vi "Longer Pump dLSP501 Operation Full Driver.vi"() -> ()   [LabVIEW 2023, in "Longer Pump dLSP501 Series.lvlib"]
uses:
  <instrlib>/Longer Pump dLSP501 Modbus RTU Series/Longer Pump dLSP501 Series.lvlib
  <vilib>/NI/Modbus Library/API/Master/Modbus Master.lvclass
  C:/Program Files/National Instruments/LabVIEW 2023/vi.lib/NI/Modbus Library/API/Modbus API.lvclass
  <instrlib>/Longer Pump dLSP501 Modbus RTU Series/Private/Initialize - Integrated Address.vi
  <vilib>/NI/Modbus Library/API/Modbus API.lvclass
panel:
  in  "Comm Port Control":cluster{"Open Port":bool, "Close Port":bool} caption="串口控制"
  in  "Operation Control":T1 caption="运行控制"
  in  "Fast Run Config":T2={"Drive Force"=80, "Run Speed"=300, "Speed Unit"="rpm", "Full Drive Force Unit"=0} caption="快速运行设置" {"Full Drive Force Unit" items=["%"]; "Run Speed" min=100 max=300 step=1; "Drive Force" min=20 max=100 step=1}
  out "Error Information":string caption="错误信息"
  out "Run Information":string caption="运行信息"
  in  "Syringe Configuration":T3={"Syringe Speicification"=1.0, "Volume Unit"=1, "Syringe Stroke"=57.1513, "Syringe Length Unit"=0} caption="注射器配置" {"Syringe Length Unit" items=["mm"]; "Syringe Stroke" min=0.001; "Volume Unit" items=["mL"=1, "uL"=2]; "Syringe Speicification" min=0.001}
  in  "Run Parameters":T4={"Run Mode"=0, "Volume Value"=1.0, "Volume Unit"=1, "Infuse Flowrate Value"=1.0, "Infuse Flowrate Unit"=1, "Withdraw Flowrate Value"=1.0, "Withdraw Flowrate Unit"=1, "Interval Time 1 Value"=1.0, "Interval Time 1 Unit"=2, "Interval Time 2 Value"=1.0, "Interval Time 2 Unit"=2, "Drive Force"=100, "Drive Force Unit"=0, "Dispensing Times"=1, "Cycles"=1} caption="运行参数" {"Drive Force Unit" items=["%"]; "Dispensing Times" min=1 max=9999; "Interval Time 2 Unit" items=["h", "min", "s"]; "Interval Time 1 Unit" items=["h", "min", "s"]; "Interval Time 2 Value" min=0.001; "Interval Time 1 Value" min=0.001; "Run Mode" items=["灌注模式", "抽取模式", "灌注/抽取模式", "抽取/灌注模式"]; "Withdraw Flowrate Unit" items=["L/min", "mL/min", "uL/min", "nL/min"]; "Withdraw Flowrate Value" min=0.001; "Infuse Flowrate Unit" items=["L/min", "mL/min", "uL/min", "nL/min"]; "Infuse Flowrate Value" min=0.001; "Volume Unit" items=["L", "mL", "uL", "nL"]; "Volume Value" min=0.001}
  out "Error out":errorcluster caption="错误输出"
  in  "Comm Config.":T5={"Address"=1, "Baud Rate"=115200, "Parity"=0} caption="通讯设置" {"Parity" items=["无校验", "奇校验", "偶校验", "标记", "空格"]; "Baud Rate" items=["1200"=1200, "2400"=2400, "9600"=9600, "19200"=19200, "38400"=38400, "57600"=57600, "115200"=115200]}
  in  "VISA resource name":refnum<visa-resource-name>="COM1" caption="VISA资源名"
  in  "Error in":errorcluster caption="错误输入"
  # "设置串口参数后，打开串口，然后进行运行控制。\n1. 全速运行；或设置运行参数、然后启动运行。\n2. 系统定期更新运行状态。"
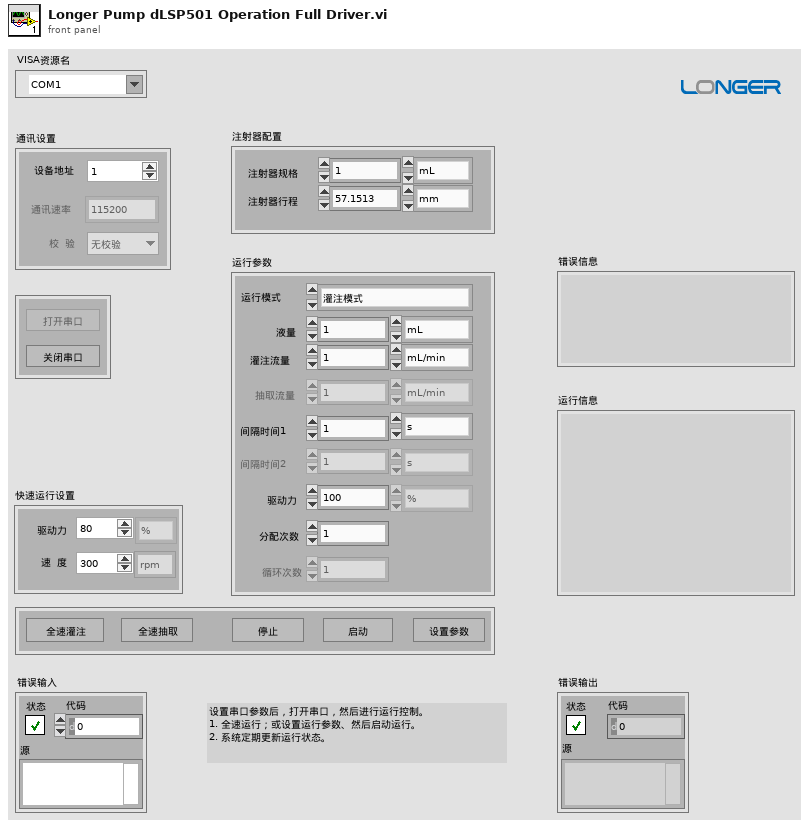
[diagram p1: front panel]
types:
  T1 = cluster{"Set Run Param":bool, "Start Run":bool, "Stop Run":bool, "Fast Infuse":bool, "Fast Withdraw":bool}
  T2 = cluster{"Drive Force":u16, "Run Speed":u16, "Speed Unit":string, "Full Drive Force Unit":u16}
  T3 = cluster{"Syringe Speicification":dbl, "Volume Unit":u16, "Syringe Stroke":dbl, "Syringe Length Unit":u16}
  T4 = cluster{"Run Mode":u16, "Volume Value":dbl, "Volume Unit":u16, "Infuse Flowrate Value":dbl, "Infuse Flowrate Unit":u16, "Withdraw Flowrate Value":dbl, "Withdraw Flowrate Unit":u16, "Interval Time 1 Value":dbl, "Interval Time 1 Unit":u16, "Interval Time 2 Value":dbl, "Interval Time 2 Unit":u16, "Drive Force":u16, "Drive Force Unit":u16, "Dispensing Times":u16, "Cycles":u16}
  T5 = cluster{"Address":u8, "Baud Rate":u32, "Parity":u16}
  T6 = enum8{"Enabled", "Disabled", "Disabled and Grayed Out"}
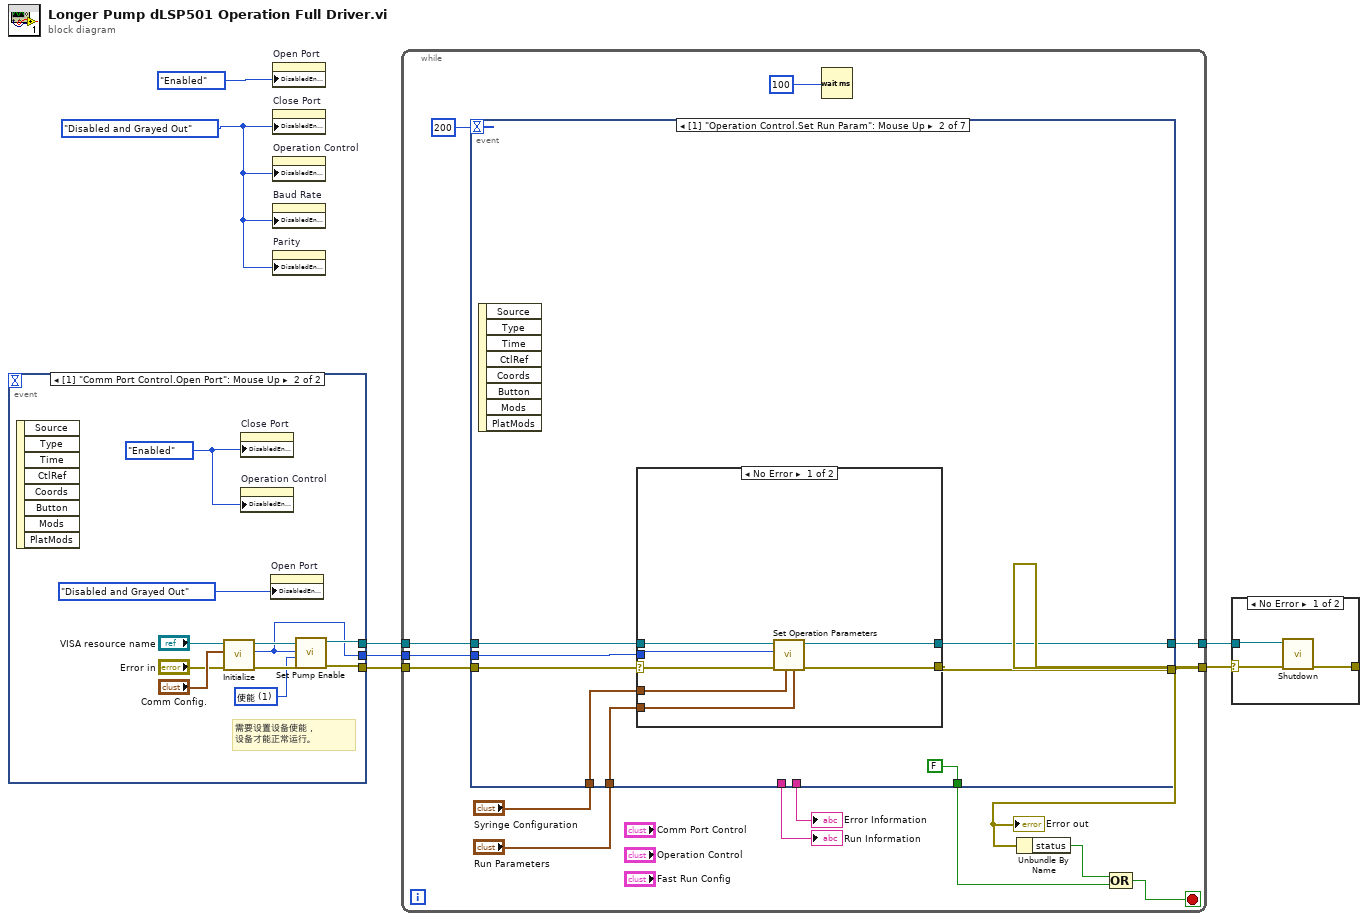
[diagram p0: block diagram]
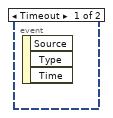
[diagram p2: hidden frame]
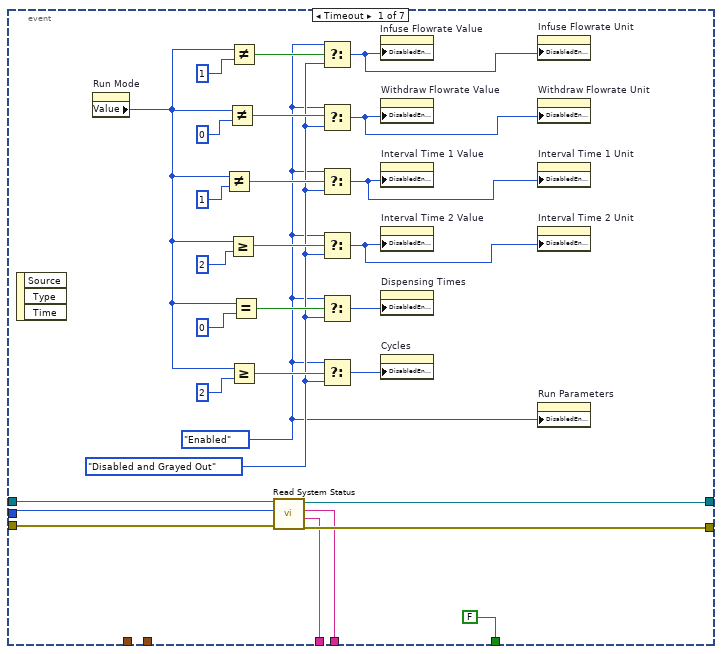
[diagram p4: hidden frame]
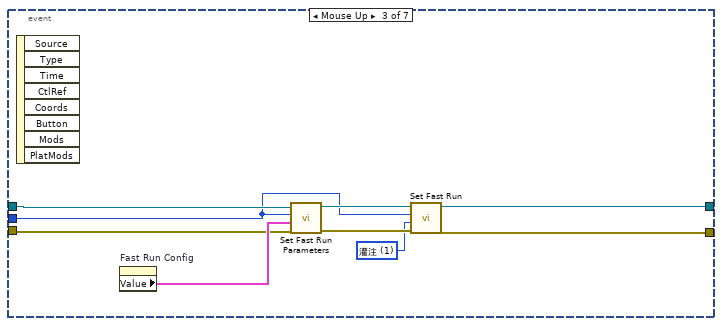
[diagram p6: hidden frame]
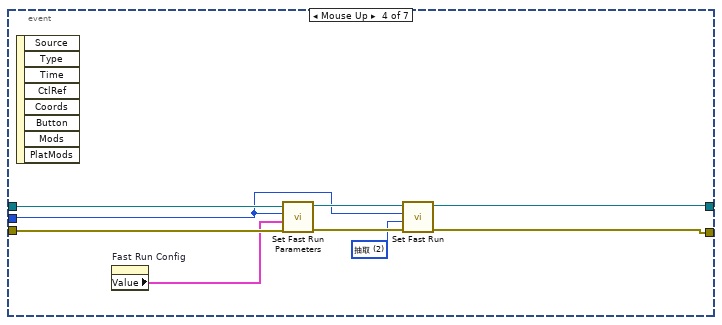
[diagram p7: hidden frame]
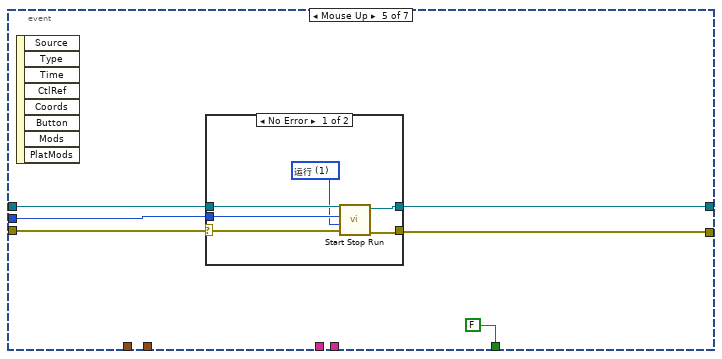
[diagram p8: hidden frame]
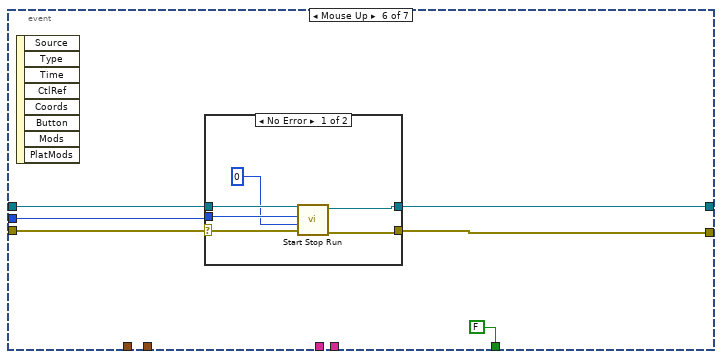
[diagram p10: hidden frame]
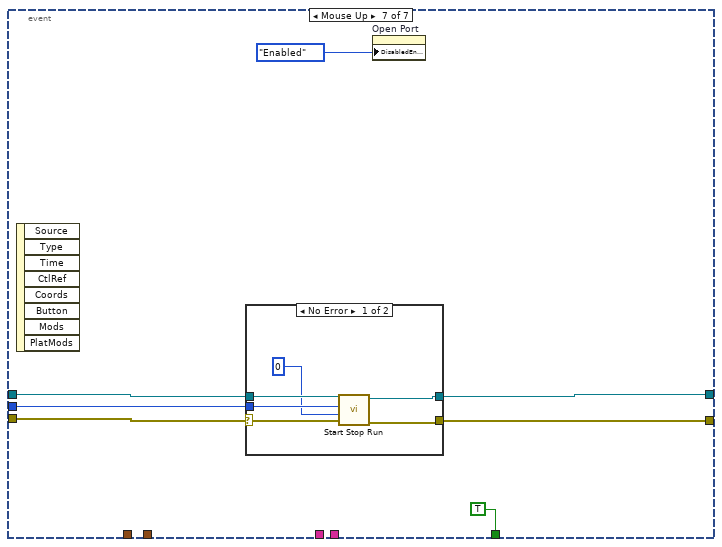
[diagram p12: hidden frame]
diagram:
  w1 = T6."Disabled and Grayed Out" ("禁用")
  n1 = event shown="[1] \"Comm Port Control.Open Port\": Mouse Up" {
    selector: _ -> [_ _]
    dyn-events: _ -> [_ _]
    timeout: _ -> [_ _]
    tunnel: [_ w12] -> w5
    tunnel: [_ w9] -> w4
    tunnel: [_ w11] -> w3
    event Timeout {
      n2 = event-data() -> ()  [unwired: 1 in, 3 out]
    }
    event "Comm Port Control.Open Port": Mouse Up {
      w10 = u16 1 items=["禁止", "使能"] ("Enable")
      w8 = T6."Enabled" ("禁用")
      # "需要设置设备使能，\n设备才能正常运行。"
      n3 = event-data() -> ()  [unwired: 1 in, 8 out]
      n4 = call-poly <instrlib>:"Initialize.vi"("Error in"="Error in", "Comm. Config"="Comm Config.", "VISA resource name"="VISA resource name") -> ("Error out"=w13:errorcluster, "Channel"=w9:i32, "serial master instance"=w14:refnum<class "Modbus Master.lvclass">)  [unwired: 5 in]
      n5 = property on="Close Port" class="Bool"("DisabledEnum"=w8) -> ()  [unwired: 2 in, 2 out]
      n6 = property on="Operation Control" class="Clust"("DisabledEnum"=w8) -> ()  [unwired: 2 in, 2 out]
      n7 = property on="Open Port" class="Bool"("DisabledEnum"=T6."Disabled and Grayed Out" ("禁用")) -> ()  [unwired: 2 in, 2 out]
      n8 = call <instrlib>:"Set Pump Enable.vi"("Error in"=w13, "Enable"=w10, "Channel"=w9, "Modbus instance in"=w14) -> ("Error out"=w12:errorcluster, "Modbus instance out"=w11:refnum<class "Modbus Master.lvclass">)  [unwired: 6 in]
    }
  }
  n9 = property on="Open Port" class="Bool"("DisabledEnum"=T6."Enabled" ("禁用")) -> ()  [unwired: 2 in, 2 out]
  n10 = property on="Close Port" class="Bool"("DisabledEnum"=w1) -> ()  [unwired: 2 in, 2 out]
  n11 = property on="Operation Control" class="Clust"("DisabledEnum"=w1) -> ()  [unwired: 2 in, 2 out]
  n12 = property on="Baud Rate" class="Ring (strict)"("DisabledEnum"=w1) -> ()  [unwired: 2 in, 2 out]
  n13 = property on="Parity" class="Ring (strict)"("DisabledEnum"=w1) -> ()  [unwired: 2 in, 2 out]
  n14 = while {
    tunnel: [w25] -> w7
    tunnel: [w30] -> w6
    tunnel: w5 -> [w27]
    tunnel: w3 -> [w29]
    tunnel: w4 -> [w28]
    stop <- w32 stop-if-true
    n15 = event shown="[1] \"Operation Control.Set Run Param\": Mouse Up" {
      selector: _ -> [_ _ _ _ _ _ _]
      dyn-events: _ -> [_ _ _ _ _ _ _]
      timeout: 200 -> [_ _ _ _ _ _ _]
      tunnel: w27 -> [w60 w65 w81 w95 w102 w114 w131]
      tunnel: w29 -> [w61 w69 w83 w96 w100 w116 w130]
      tunnel: [w57 w68 w79 w94 w99 w112 w129] -> w30
      tunnel: [w58 w67 w80 w93 w98 w113 w128] -> w25
      tunnel: w28 -> [w59 w66 w82 w90 w101 w115 w127]
      tunnel: [w56 _ _ _ _ _ _] -> w24
      tunnel: [w55 _ _ _ _ _ _] -> w23
      tunnel: "Run Parameters" -> [_ w64 _ _ _ _ _]
      tunnel: "Syringe Configuration" -> [_ w63 _ _ _ _ _]
      tunnel: [FALSE FALSE _ _ FALSE FALSE TRUE] -> w19
      event Timeout {
        w36 = T6."Disabled and Grayed Out" ("禁用")
        w34 = T6."Enabled" ("禁用")
        n16 = event-data() -> ()  [unwired: 1 in, 3 out]
        n17 = property on="Run Mode" class="Ring (strict)"() -> ("Value"=w35:u16)  [unwired: 2 in, 2 out]
        n18 = Not Equal?(x=w35, y=u16 1) -> (x != y?=w48:bool)
        n19 = Not Equal?(x=w35, y=u16 0) -> (x != y?=w45:bool)
        n20 = Greater Or Equal?(x=w35, y=u16 2) -> (x >= y?=w53:bool)
        n21 = Not Equal?(x=w35, y=u16 1) -> (x != y?=w46:bool)
        n22 = Greater Or Equal?(x=w35, y=u16 2) -> (x >= y?=w54:bool)
        n23 = Equal?(x=w35, y=u16 0) -> (x = y?=w43:bool)
        n24 = call <instrlib>:"Read System Status.vi"("Error in"=w60, "Channel"=w59, "Modbus master in"=w61) -> ("Error out"=w58:errorcluster, "Run Status Information"=w55:string, "Error Information"=w56:string, "Modbus instance out"=w57:refnum<class "Modbus API.lvclass">)  [unwired: 5 in]
        n25 = Select(t=w34, s=w46, f=w36) -> (s? t:f=w49:T6)
        n26 = Select(t=w34, s=w45, f=w36) -> (s? t:f=w50:T6)
        n27 = Select(t=w34, s=w48, f=w36) -> (s? t:f=w51:T6)
        n28 = Select(t=w34, s=w53, f=w36) -> (s? t:f=w52:T6)
        n29 = Select(t=w34, s=w43, f=w36) -> (s? t:f=w44:T6)
        n30 = Select(t=w34, s=w54, f=w36) -> (s? t:f=w47:T6)
        n31 = property on="Infuse Flowrate Value" class="DigNum (strict)"("DisabledEnum"=w49) -> ()  [unwired: 2 in, 2 out]
        n32 = property on="Withdraw Flowrate Value" class="DigNum (strict)"("DisabledEnum"=w50) -> ()  [unwired: 2 in, 2 out]
        n33 = property on="Interval Time 1 Value" class="DigNum (strict)"("DisabledEnum"=w51) -> ()  [unwired: 2 in, 2 out]
        n34 = property on="Interval Time 2 Value" class="DigNum (strict)"("DisabledEnum"=w52) -> ()  [unwired: 2 in, 2 out]
        n35 = property on="Dispensing Times" class="DigNum (strict)"("DisabledEnum"=w44) -> ()  [unwired: 2 in, 2 out]
        n36 = property on="Cycles" class="DigNum (strict)"("DisabledEnum"=w47) -> ()  [unwired: 2 in, 2 out]
        n37 = property on="Infuse Flowrate Unit" class="Ring (strict)"("DisabledEnum"=w49) -> ()  [unwired: 2 in, 2 out]
        n38 = property on="Withdraw Flowrate Unit" class="Ring (strict)"("DisabledEnum"=w50) -> ()  [unwired: 2 in, 2 out]
        n39 = property on="Interval Time 1 Unit" class="Ring (strict)"("DisabledEnum"=w51) -> ()  [unwired: 2 in, 2 out]
        n40 = property on="Interval Time 2 Unit" class="Ring (strict)"("DisabledEnum"=w52) -> ()  [unwired: 2 in, 2 out]
        n41 = property on="Run Parameters" class="Clust (strict)"("DisabledEnum"=w34) -> ()  [unwired: 2 in, 2 out]
      }
      event "Operation Control.Set Run Param": Mouse Up {
        n42 = event-data() -> ()  [unwired: 1 in, 8 out]
        n43 = case shown="No Error" w65 {
          selector: w65 -> [w72 w77]
          tunnel: w69 -> [w73 w78]
          tunnel: [w76 w78] -> w68
          tunnel: [w75 w77] -> w67
          tunnel: w64 -> [w70 _]
          tunnel: w66 -> [w74 _]
          tunnel: w63 -> [w71 _]
          frame No Error {
            n44 = call <instrlib>:"Set Operation Parameters.vi"("Run Parameters"=w70, "Syringe Configuration"=w71, "Error in"=w72, "Channel"=w74, "Modbus master in"=w73) -> ("Error out"=w75:errorcluster, "Modbus instance out"=w76:refnum<class "Modbus API.lvclass">)  [unwired: 5 in]
          }
          frame Error {
          }
        }
      }
      event "Operation Control.Fast Infuse": Mouse Up {
        w84 = u16 1 items=["停止", "灌注", "抽取"] ("Full Speed Control")
        n45 = event-data() -> ()  [unwired: 1 in, 8 out]
        n46 = property on="Fast Run Config" class="Clust (strict)"() -> ("Value"=w87:T2)  [unwired: 2 in, 2 out]
        n47 = call <instrlib>:"Set Fast Run Parameters.vi"("Error in"=w81, "Full Speed Config"=w87, "Channel"=w82, "Modbus instance in"=w83) -> ("Error out"=w85:errorcluster, "Modbus instance out"=w86:refnum<class "Modbus Master.lvclass">)  [unwired: 6 in]
        n48 = call <instrlib>:"Set Fast Run.vi"("Error in"=w85, "Full Speed Control"=w84, "Channel"=w82, "Modbus instance in"=w86) -> ("Error out"=w80:errorcluster, "Modbus instance out"=w79:refnum<class "Modbus Master.lvclass">)  [unwired: 6 in]
      }
      event "Operation Control.Fast Withdraw": Mouse Up {
        w89 = u16 2 items=["停止", "灌注", "抽取"] ("Full Speed Control")
        n49 = event-data() -> ()  [unwired: 1 in, 8 out]
        n50 = property on="Fast Run Config" class="Clust (strict)"() -> ("Value"=w88:T2)  [unwired: 2 in, 2 out]
        n51 = call <instrlib>:"Set Fast Run Parameters.vi"("Error in"=w95, "Full Speed Config"=w88, "Channel"=w90, "Modbus instance in"=w96) -> ("Error out"=w92:errorcluster, "Modbus instance out"=w91:refnum<class "Modbus Master.lvclass">)  [unwired: 6 in]
        n52 = call <instrlib>:"Set Fast Run.vi"("Error in"=w92, "Full Speed Control"=w89, "Channel"=w90, "Modbus instance in"=w91) -> ("Error out"=w93:errorcluster, "Modbus instance out"=w94:refnum<class "Modbus Master.lvclass">)  [unwired: 6 in]
      }
      event "Operation Control.Start Run": Mouse Up {
        n53 = event-data() -> ()  [unwired: 1 in, 8 out]
        n54 = case shown="No Error" w102 {
          selector: w102 -> [w107 w109]
          tunnel: w100 -> [w108 w110]
          tunnel: [w106 w110] -> w99
          tunnel: [w105 w109] -> w98
          tunnel: w101 -> [w104 _]
          frame No Error {
            w103 = u16 1 items=["停止", "运行"] ("Start/Stop")
            n55 = call <instrlib>:"Start Stop Run.vi"("Error in"=w107, "Start/Stop"=w103, "Channel"=w104, "Modbus instance in"=w108) -> ("Error out"=w105:errorcluster, "Modbus instance out"=w106:refnum<class "Modbus Master.lvclass">)  [unwired: 6 in]
          }
          frame Error {
          }
        }
      }
      event "Operation Control.Stop Run": Mouse Up {
        n56 = event-data() -> ()  [unwired: 1 in, 8 out]
        n57 = case shown="No Error" w114 {
          selector: w114 -> [w121 w123]
          tunnel: w116 -> [w122 w124]
          tunnel: [w120 w124] -> w112
          tunnel: [w119 w123] -> w113
          tunnel: w115 -> [w118 _]
          frame No Error {
            n58 = call <instrlib>:"Start Stop Run.vi"("Error in"=w121, "Start/Stop"=0, "Channel"=w118, "Modbus instance in"=w122) -> ("Error out"=w119:errorcluster, "Modbus instance out"=w120:refnum<class "Modbus Master.lvclass">)  [unwired: 6 in]
          }
          frame Error {
          }
        }
      }
      event "Comm Port Control.Close Port": Mouse Up {
        n59 = event-data() -> ()  [unwired: 1 in, 8 out]
        n60 = case shown="No Error" w131 {
          selector: w131 -> [w136 w138]
          tunnel: w130 -> [w137 w139]
          tunnel: [w135 w139] -> w129
          tunnel: [w134 w138] -> w128
          tunnel: w127 -> [w133 _]
          frame No Error {
            n61 = call <instrlib>:"Start Stop Run.vi"("Error in"=w136, "Start/Stop"=0, "Channel"=w133, "Modbus instance in"=w137) -> ("Error out"=w134:errorcluster, "Modbus instance out"=w135:refnum<class "Modbus Master.lvclass">)  [unwired: 6 in]
          }
          frame Error {
          }
        }
        n62 = property on="Open Port" class="Bool"("DisabledEnum"=T6."Enabled" ("禁用")) -> ()  [unwired: 2 in, 2 out]
      }
    }
    "Error out" <- w25
    "Run Information" <- w23
    "Error Information" <- w24
    n63 = Wait (ms)(milliseconds to wait=u32 100 ("毫秒计时值")) -> ()  [unwired: 1 out]
    n64 = Unbundle By Name(w25) -> ("status"=w26:bool)
    n65 = Compound Arithmetic op=OR ("复合运算")(w26, w19) -> (w32:bool)
  }
  n66 = case shown="No Error" w7 {
    selector: w7 -> [w141 w143]
    tunnel: w6 -> [w142 _]
    tunnel: [w140 w143] -> _
    frame No Error {
      n67 = call-dynamic "Shutdown.vi"("error in"=w141, "Modbus instance in"=w142) -> ("error out"=w140:errorcluster)  [unwired: 9 in]
    }
    frame Error {
    }
  }
